vi "user event out.vi"() -> ()   [LabVIEW 2014]
uses:
  Move stage command.ctl
panel:
  out "user event out":refnum<user-event>
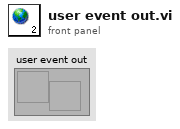
[diagram p1: front panel]
diagram:
